vi "Field Centric Test.vi"() -> ()   [LabVIEW 2020]
uses:
  <vilib>/ptbypt/NI_PtbyPt.lvlib
panel:
  in  "IMU":dbl(slide) scale=-180.0..180.0
  out "Arcade Inputs":picture
  out "XY Graph":cluster{dbl[], dbl[]}[](graph)
  # "Front (1)"
  # "Left (-1)"
  # "Right (1)"
  # "Back (-1)"
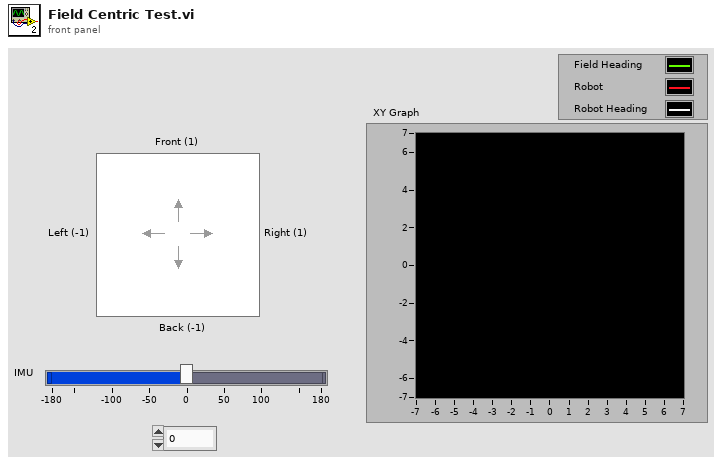
[diagram p1: front panel]
types:
  T1 = typedef "LVMouseTypeDef.ctl" = cluster{"Mouse Position":cluster{"X":i32, "Y":i32}, "Mouse Modifiers":cluster{"Button Down":bool, "Shift Mod":bool, "Menu Mod":bool, "Option Mod":bool}}
  T2 = typedef "LVBoundsTypeDef.ctl" = cluster{"Width":u32, "Height":u32}
  T3 = cluster{"Start X":dbl, "Wrapped IMU (radians)":dbl}
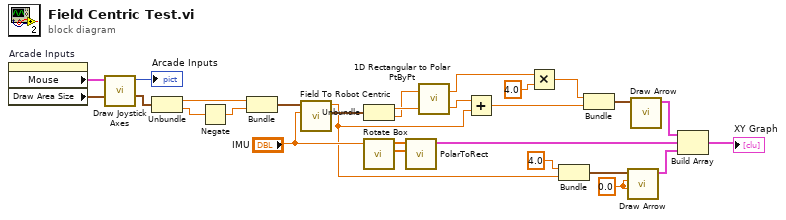
[diagram p0: block diagram]
diagram:
  w25 = 0.0 ("Start X")
  n1 = property on="Arcade Inputs" class="Pict"() -> ("Mouse"=w27:T1, "Draw Area Size"=w18:T2)  [unwired: 2 in, 2 out]
  n2 = call "Draw Joystick Axes.vi"("Size"=w18, "Mouse"=w27) -> ("JS Coords"=w26:cluster{"X":dbl, "Y":dbl}, "Arcade Inputs"=→"Arcade Inputs":picture)  [unwired: 8 in]
  n3 = Unbundle(w26) -> ("X"=w5:dbl, "Y"=w11:dbl)
  n4 = Negate(x=w11) -> (-x=w6:dbl)
  n5 = Bundle("X"=w5, w6) -> (w4:cluster{"X":dbl, dbl})  [unwired: 1 in]
  n6 = call "Field To Robot Centric.vi"("IMU Value (offset)"="IMU", "Translation Joystick"=w4) -> ("Robot Centric Vector"=w2:cluster{dbl, dbl}, "Wrapped IMU (radians)"=w1:dbl)  [unwired: 8 in]
  n7 = Unbundle(w2) -> (w15:dbl, w14:dbl)
  n8 = call "Rotate Box.vi"("IMU"="IMU") -> ("theta"=w24:dbl[], "r"=w23:dbl[])  [unwired: 7 in]
  n9 = call "PolarToRect.vi"("theta"=w24, "r"=w23) -> ("Rectangular Coordinates"=w20:cluster{dbl[], dbl[]})  [unwired: 9 in]
  n10 = call <vilib>:"1D Rectangular to Polar PtByPt.vi"("y"=w15, "x"=w14) -> ("phase"=w13:dbl, "magnitude"=w10:dbl)
  n11 = Add(x=w13, y=w1) -> (x+y=w12:dbl)
  n12 = Multiply(x=w10, y=4.0) -> (x*y=w8:dbl)
  n13 = Bundle("Start X"=4.0, "Wrapped IMU (radians)"=w1) -> (w17:T3)  [unwired: 1 in]
  n14 = Bundle(w8, w12) -> (w7:cluster{dbl, dbl})  [unwired: 1 in]
  n15 = call "Draw Arrow.vi"("Start Y"=w25, "Start X"=w25, "Vector"=w17) -> ("Points"=w21:cluster{dbl[], dbl[]})  [unwired: 6 in, 2 out]
  n16 = call "Draw Arrow.vi"("Vector"=w7) -> ("Points"=w16:cluster{dbl[], dbl[]})  [unwired: 8 in, 2 out]
  n17 = Build Array(w16, w20, w21) -> (→"XY Graph":cluster{dbl[], dbl[]}[])
